vi "TestApplymain.vi"() -> ()   [LabVIEW 2021]
uses:
  <vilib>/Instr/_visa.llb/VISA Configure Serial Port (Instr).vi
panel:
  in  "stop":bool
  in  "Bouton OFFSET":bool
  in  "VISA resource name":refnum<visa-resource-name> caption="PORT DSCUSB"
  in  "Bouton Parametre":bool
  out "buffer de lecture":string
  out "Poids sur le capteur":dbl
  out "Alarme":bool
  in  "Chaîne déroulante":string(combo)
  out "Graphe déroulant":dbl(graph)
  in  "Enregister":bool
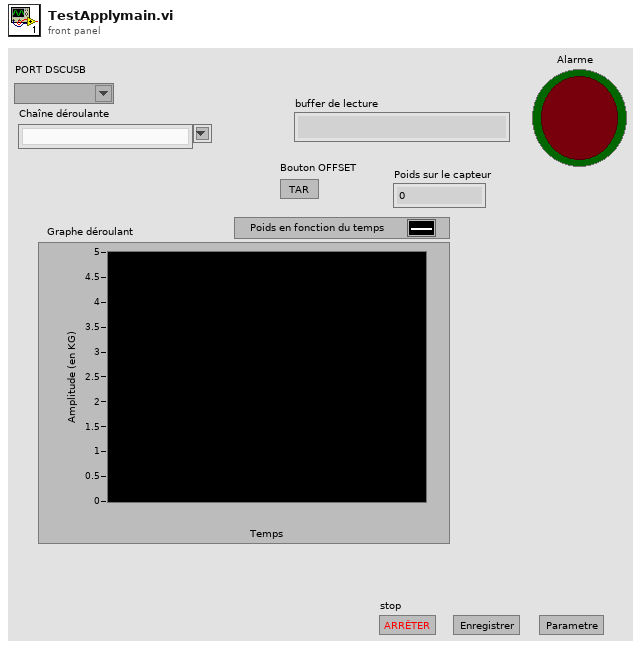
[diagram p1: front panel]
types:
  T1 = enum16{"open", "replace", "create", "open or create", "replace or create", "replace or create with confirmation"}
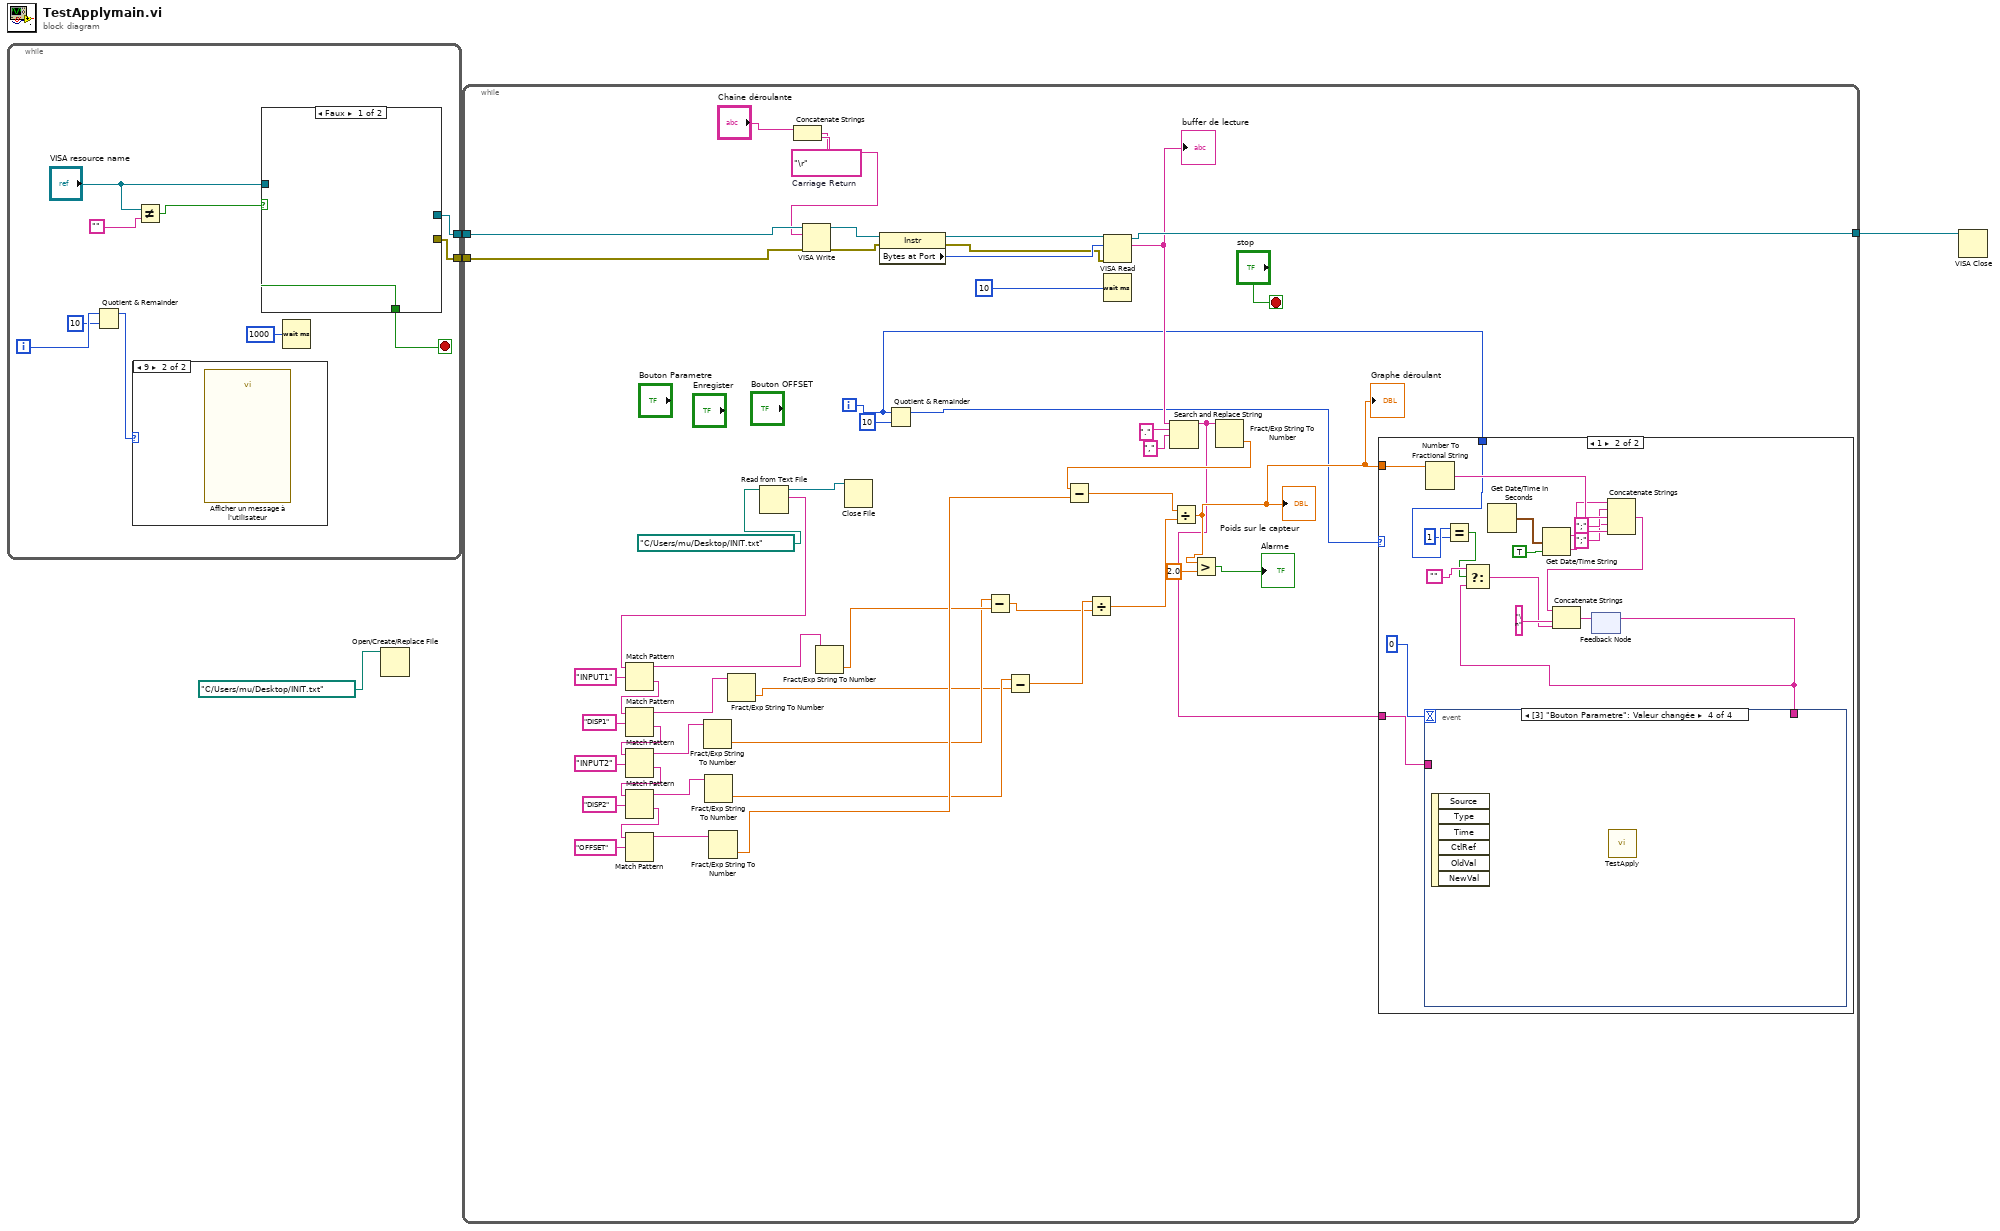
[diagram p0: block diagram]
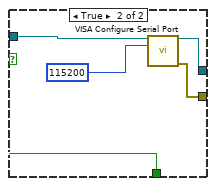
[diagram p3: hidden frame]
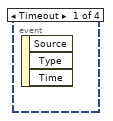
[diagram p5: hidden frame]
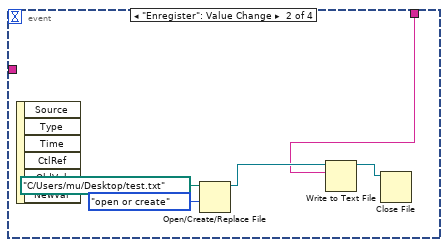
[diagram p6: hidden frame]
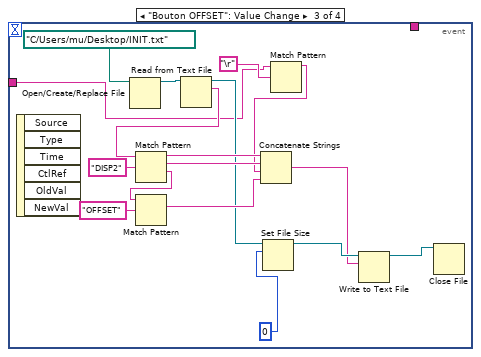
[diagram p7: hidden frame]
diagram:
  n1 = while {
    tunnel: [w14] -> w3
    tunnel: [w13] -> w2
    i -> [w7]
    stop <- w8 stop-if-true
    n2 = Quotient & Remainder(x=w7, y=10) -> (x-y*floor(x/y)=w5:i32)  [unwired: 1 out]
    n3 = case shown="9" w5 {
      frame 0, Default {
      }
      frame 9 {
        n4 = call "Afficher un message à l'utilisateur"() -> ()  [unwired: 10 in, 2 out]
      }
    }
    n5 = Not Equal?(x="VISA resource name", y="") -> (x != y?=w10:bool)
    n6 = case shown="Faux" w10 {
      selector: w10 -> [w15 w16]
      tunnel: "VISA resource name" -> [_ w19]
      tunnel: [_ w18] -> w14
      tunnel: [_ w17] -> w13
      tunnel: [w15 w16] -> w8
      frame False {
      }
      frame True {
        n7 = call-poly "VISA Configure Serial Port"("VISA resource name"=w19, "baud rate (9600)"=u32 115200) -> ("VISA resource name out"=w18:refnum<visa-resource-name>, "error out"=w17:errorcluster)  [unwired: 12 in]
      }
    }
    n8 = Wait (ms)(milliseconds to wait=u32 1000 ("attente (ms)")) -> ()  [unwired: 1 out]
  }
  n9 = Open/Create/Replace File(file path (use dialog)=path "C:/Users/mu/Desktop/INIT.txt" ("chemin du fichier (utiliser une boîte de dialogue)")) -> ()  [unwired: 5 in, 3 out]
  n10 = while {
    tunnel: w3 -> [w70]
    tunnel: w2 -> [w69]
    tunnel: [w63] -> w4
    i -> [w23]
    stop <- "stop" stop-if-true
    w62 = "\r"  # Carriage Return
    n11 = Read from Text File(file (use dialog)=path "C:/Users/mu/Desktop/INIT.txt" ("fichier (utiliser une boîte de dialogue)")) -> (refnum out=w24:refnum<file>, text=w50:string)  [unwired: 3 in, 2 out]
    n12 = Match Pattern(string=w50, regular expression="INPUT1" ("expression régulière")) -> (before substring=w36:string, after substring=w46:string)  [unwired: 1 in, 2 out]
    n13 = Match Pattern(string=w46, regular expression="DISP1" ("expression régulière")) -> (before substring=w37:string, after substring=w47:string)  [unwired: 1 in, 2 out]
    n14 = Match Pattern(string=w47, regular expression="INPUT2" ("expression régulière")) -> (before substring=w38:string, after substring=w48:string)  [unwired: 1 in, 2 out]
    n15 = Match Pattern(string=w48, regular expression="DISP2" ("expression régulière")) -> (before substring=w39:string, after substring=w49:string)  [unwired: 1 in, 2 out]
    n16 = Match Pattern(string=w49, regular expression="OFFSET" ("expression régulière")) -> (before substring=w40:string)  [unwired: 1 in, 3 out]
    n17 = Fract/Exp String To Number(string=w38) -> (number=w32:dbl)  [unwired: 3 in, 1 out]
    n18 = Fract/Exp String To Number(string=w39) -> (number=w31:dbl)  [unwired: 3 in, 1 out]
    n19 = Fract/Exp String To Number(string=w40) -> (number=w34:dbl)  [unwired: 3 in, 1 out]
    n20 = Fract/Exp String To Number(string=w37) -> (number=w30:dbl)  [unwired: 3 in, 1 out]
    n21 = Concatenate Strings("Chaîne déroulante", w62) -> (w61:string)
    n22 = VISA Write(VISA resource name=w70, write buffer=w61, error in (no error)=w69) -> (VISA resource name out=w68:refnum<visa-resource-name>, error out=w67:errorcluster)  [unwired: 1 out]
    n23 = Fract/Exp String To Number(string=w36) -> (number=w33:dbl)  [unwired: 3 in, 1 out]
    n24 = Close File(refnum=w24) -> ()  [unwired: 1 in, 2 out]
    n25 = property class="Instr"(reference=w68, error in=w67) -> (reference out=w66:refnum<visa-resource-name>, error out=w64:errorcluster, "Bytes at Port"=w65:u32)
    n26 = Quotient & Remainder(x=w23, y=10) -> (x-y*floor(x/y)=w51:i32)  [unwired: 1 out]
    n27 = Subtract(x=w32, y=w33) -> (x-y=w28:dbl)
    n28 = Subtract(x=w31, y=w30) -> (x-y=w29:dbl)
    n29 = Divide(x=w29, y=w28) -> (x/y=w27:dbl)
    n30 = VISA Read(VISA resource name=w66, byte count=w65, error in (no error)=w64) -> (VISA resource name out=w63:refnum<visa-resource-name>, read buffer=w57:string)  [unwired: 2 out]
    "buffer de lecture" <- w57
    n31 = Wait (ms)(milliseconds to wait=u32 10 ("attente (ms)")) -> ()  [unwired: 1 out]
    n32 = Search and Replace String(input string=w57, search string=".", replace string=",") -> (result string=w25:string)  [unwired: 5 in, 3 out]
    n33 = Fract/Exp String To Number(string=w25) -> (number=w35:dbl)  [unwired: 3 in, 1 out]
    n34 = Subtract(x=w35, y=w34) -> (x-y=w26:dbl)
    n35 = Divide(x=w26, y=w27) -> (x/y=w53:dbl)
    "Poids sur le capteur" <- w53
    "Graphe déroulant" <- w53
    n36 = Greater?(x=w53, y=2.0) -> (0:→"Alarme":bool)
    n37 = case shown="1" w51 {
      tunnel: w53 -> [_ w89]
      tunnel: w23 -> [_ w73]
      tunnel: w25 -> [_ w75]
      frame 0, Default {
      }
      frame 1 {
        n38 = Number To Fractional String(number=w89) -> (F-format string=w87:string)  [unwired: 3 in]
        n39 = Equal?(x=w73, y=1) -> (x = y?=w71:bool)
        n40 = Get Date/Time In Seconds() -> (seconds since 1Jan1904=w88:timestamp)
        n41 = Get Date/Time String(seconds (now)=w88, want seconds? (F)=TRUE ("secondes ? (F)")) -> (date string=w86:string, time string=w85:string)  [unwired: 1 in]
        n42 = feedback #1() -> (w74:string)  [unwired: 1 in]
        n43 = event shown="[3] \"Bouton Parametre\": Valeur changée" {
          selector: _ -> [_ _ _ _]
          dyn-events: _ -> [_ _ _ _]
          timeout: 0 -> [_ _ _ _]
          tunnel: w74 -> [_ w93 _ _]
          tunnel: w75 -> [_ _ w95 _]
          event Timeout {
            n44 = event-data() -> ()  [unwired: 1 in, 3 out]
          }
          event "Enregister": Value Change {
            n45 = event-data() -> ()  [unwired: 1 in, 6 out]
            n46 = Open/Create/Replace File(file path (use dialog)=path "C:/Users/mu/Desktop/test.txt" ("chemin du fichier (utiliser une boîte de dialogue)"), operation (0:open)=T1."open or create" ("opération (0 : open)")) -> (refnum out=w94:refnum<file>)  [unwired: 4 in, 2 out]
            n47 = Write to Text File(file (use dialog)=w94, text=w93) -> (refnum out=w92:refnum<file>)  [unwired: 2 in, 2 out]
            n48 = Close File(refnum=w92) -> ()  [unwired: 1 in, 2 out]
          }
          event "Bouton OFFSET": Value Change {
            n49 = event-data() -> ()  [unwired: 1 in, 6 out]
            n50 = Open/Create/Replace File(file path (use dialog)=path "C:/Users/mu/Desktop/INIT.txt" ("chemin du fichier (utiliser une boîte de dialogue)")) -> (refnum out=w110:refnum<file>)  [unwired: 5 in, 2 out]
            n51 = Read from Text File(file (use dialog)=w110) -> (refnum out=w97:refnum<file>, text=w109:string)  [unwired: 3 in, 2 out]
            n52 = Match Pattern(string=w109, regular expression="DISP2" ("expression régulière")) -> (before substring=w108:string, match substring=w107:string, after substring=w105:string)  [unwired: 1 in, 1 out]
            n53 = Match Pattern(string=w105, regular expression="OFFSET" ("expression régulière")) -> (match substring=w103:string)  [unwired: 1 in, 3 out]
            n54 = Set File Size(6:i64 0 ("taille (en octets)"), 7:w97) -> (3:w100:refnum<file>)  [unwired: 1 in, 1 out]
            n55 = Match Pattern(string=w95, regular expression="\r") -> (before substring=w101:string)  [unwired: 1 in, 3 out]
            n56 = Concatenate Strings(w108, w107, w101, w103) -> (w96:string)
            n57 = Write to Text File(file (use dialog)=w100, text=w96) -> (refnum out=w99:refnum<file>)  [unwired: 2 in, 2 out]
            n58 = Close File(refnum=w99) -> ()  [unwired: 1 in, 2 out]
          }
          event "Bouton Parametre": Value Change {
            n59 = event-data() -> ()  [unwired: 1 in, 6 out]
            n60 = call "TestApply.vi"() -> ()  [unwired: 12 in]
          }
        }
        n61 = Select(t="", s=w71, f=w74) -> (s? t:f=w77:string)
        n62 = Concatenate Strings(w86, ";" ("chaîne"), w85, ";" ("chaîne"), w87) -> (w79:string)
        n63 = Concatenate Strings(w79, "\n" ("chaîne"), w77) -> (w78:string)
        n64 = feedback-in #1(w78) -> ()
      }
    }
  }
  n65 = VISA Close(VISA resource name=w4) -> ()  [unwired: 1 in, 1 out]
